vi "Basic Function Return Value.vi"() -> ()   [LabVIEW 2014]
panel:
  out "Error Out":errorcluster
  in  "Error In":errorcluster
  out "resulting string":string
  in  "return variable name":string
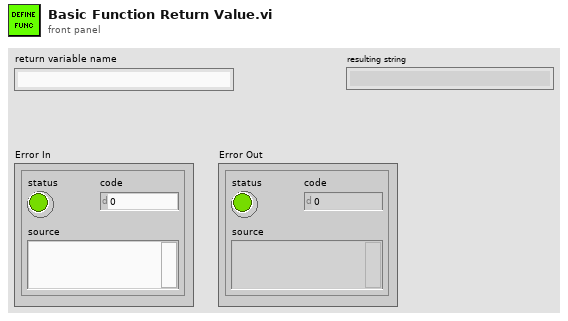
[diagram p1: front panel]
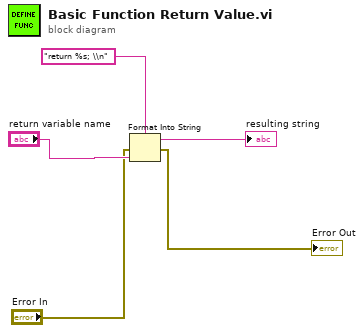
[diagram p0: block diagram]
diagram:
  n1 = Format Into String(format string="return %s; \\n", error in="Error In", "return variable name") -> (resulting string=→"resulting string":string, error out=→"Error Out":errorcluster)  [unwired: 1 in]
